vi "Panel Object Settings Changed.vi"(8 "Error In":errorcluster, 11 "Pane Relief Main UI in":refnum<class "Pane Relief Main UI.lvclass">) -> (0 "Error Out":errorcluster, 3 "Pane Relief Main UI out":refnum<class "Pane Relief Main UI.lvclass">)   [LabVIEW 2017, in "Pane Relief Main UI.lvlib" / "Pane Relief Main UI.lvclass"]
uses:
  Pane Relief Main UI.lvclass
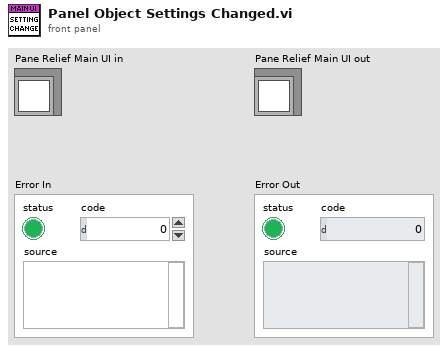
[diagram p1: front panel]
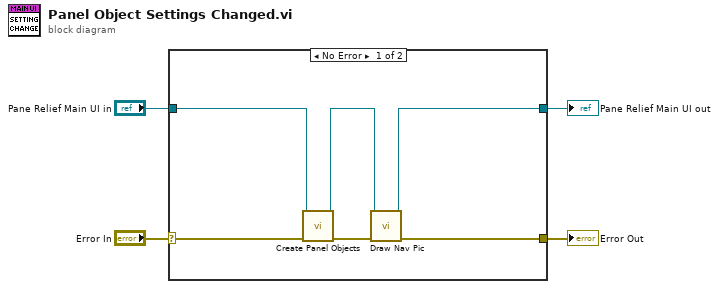
[diagram p0: block diagram]
diagram:
  n1 = case shown="No Error" "Error In" {
    selector: "Error In" -> [w10 w12]
    tunnel: [w9 w12] -> w1
    tunnel: [w6 w11] -> w3
    tunnel: "Pane Relief Main UI in" -> [w7 w11]
    frame No Error {
      n2 = call-dynamic "Create Panel Objects.vi"("Error In"=w10, "Pane Relief Main UI in"=w7) -> ("Error Out"=w5:errorcluster, "Pane Relief Main UI out"=w8:refnum<class "Pane Relief Main UI.lvclass">)  [unwired: 8 in]
      n3 = call-dynamic "Draw Nav Pic.vi"("Error In"=w5, "Pane Relief Main UI in"=w8) -> ("Error Out"=w9:errorcluster, "Pane Relief Main UI out"=w6:refnum<class "Pane Relief Main UI.lvclass">)  [unwired: 8 in]
    }
    frame Error {
    }
  }
  "Pane Relief Main UI out" <- w3
  "Error Out" <- w1
